vi "Check_Value_Range.vi"(1 "Min":sgl, 2 "Data in":sgl caption="Numeric", 3 "Max":sgl) -> (0 "Data out":sgl caption="Numeric")   [LabVIEW 2012]
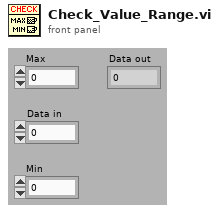
[diagram p1: front panel]
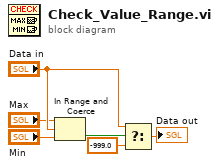
[diagram p0: block diagram]
diagram:
  n1 = In Range and Coerce(upper limit="Max", x="Data in", lower limit="Min") -> (In Range?=w6:bool)  [unwired: 1 out]
  n2 = Select(t="Data in", s=w6, f=sgl -999.0) -> (s? t:f=→"Data out":sgl)
